vi "ProjetoTASCA.vi"(11 "Measurement Time (s)":sgl=1.0) -> (1 "Coincidences":u32=9, 2 "Count 1":u32=42663, 3 "Count 0":u32=44178)   [LabVIEW 2013]
uses:
  <vilib>/eio/EIONode/EIONode.xnode
  <vilib>/rvi/eio/common/nirviEmuTemplateMethod_errors.vi
  <vilib>/Platform/TimedLoop/XDataNode/XDataNode.xnode
  <vilib>/Platform/TimedLoop/XDataNode/timing_clust.ctl
  <vilib>/Platform/TimedLoop/XDataNode/XDNodeRunTimeDep.lvlib
  <vilib>/Platform/TimedLoop/XDataNode/wakeup.ctl
  <vilib>/Platform/TimedLoop/XDataNode/nitl_modes.ctl
panel:
  out "execution rate out":u32
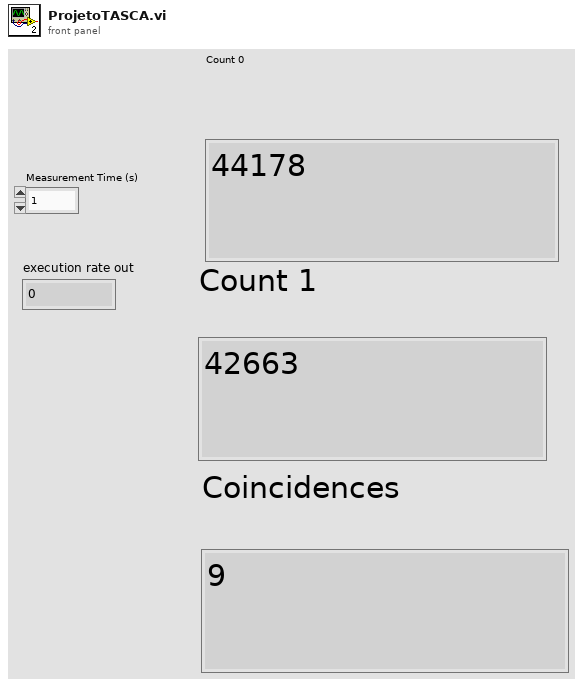
[diagram p1: front panel]
types:
  T1 = typedef "XDNodeRunTimeDep.lvlib/timing_clust.ctl" = cluster{"Expected End [f-1]":u64, "Actual End [f-1]":u64, "Finished Late? [f-1]":bool, "Expected End [i-1]":u64, "Actual End [i-1]":u64, "Finished Late? [i-1]":bool, "Expected Start [i]":u64, "Actual Start [i]":u64, "Expected Start [f]":u64, "Actual Start [f]":u64, "Source Name":string, "Structure Name":string, "Period":i64, "Deadline":i64, "Offset":i64, "Start":i64, "Priority":i32, "Timeout":i32, "Mode":T2, "Wakeup Reason":T3, "Error":errorcluster, "Source Type":string, "Secondary Source Type":string, "Global End Time":u64, "Global Start Time":u64, "Frame Duration":u64, "Iteration Duration":u64, "Assigned CPU":i32, "I/O Scan Engine Mode":u32}
  T2 = typedef "XDNodeRunTimeDep.lvlib/nitl_modes.ctl" = enum32{"No Change", "Process missed periods, maintain original phase", "Discard missed periods, maintain original phase", "Process missed periods, ignore original phase", "Discard missed periods, ignore original phase"}
  T3 = typedef "XDNodeRunTimeDep.lvlib/wakeup.ctl" = enum32{"Normal", "Aborted", "Asynchronous wakeup", "Timing source error", "Timed loop error", "Timeout"}
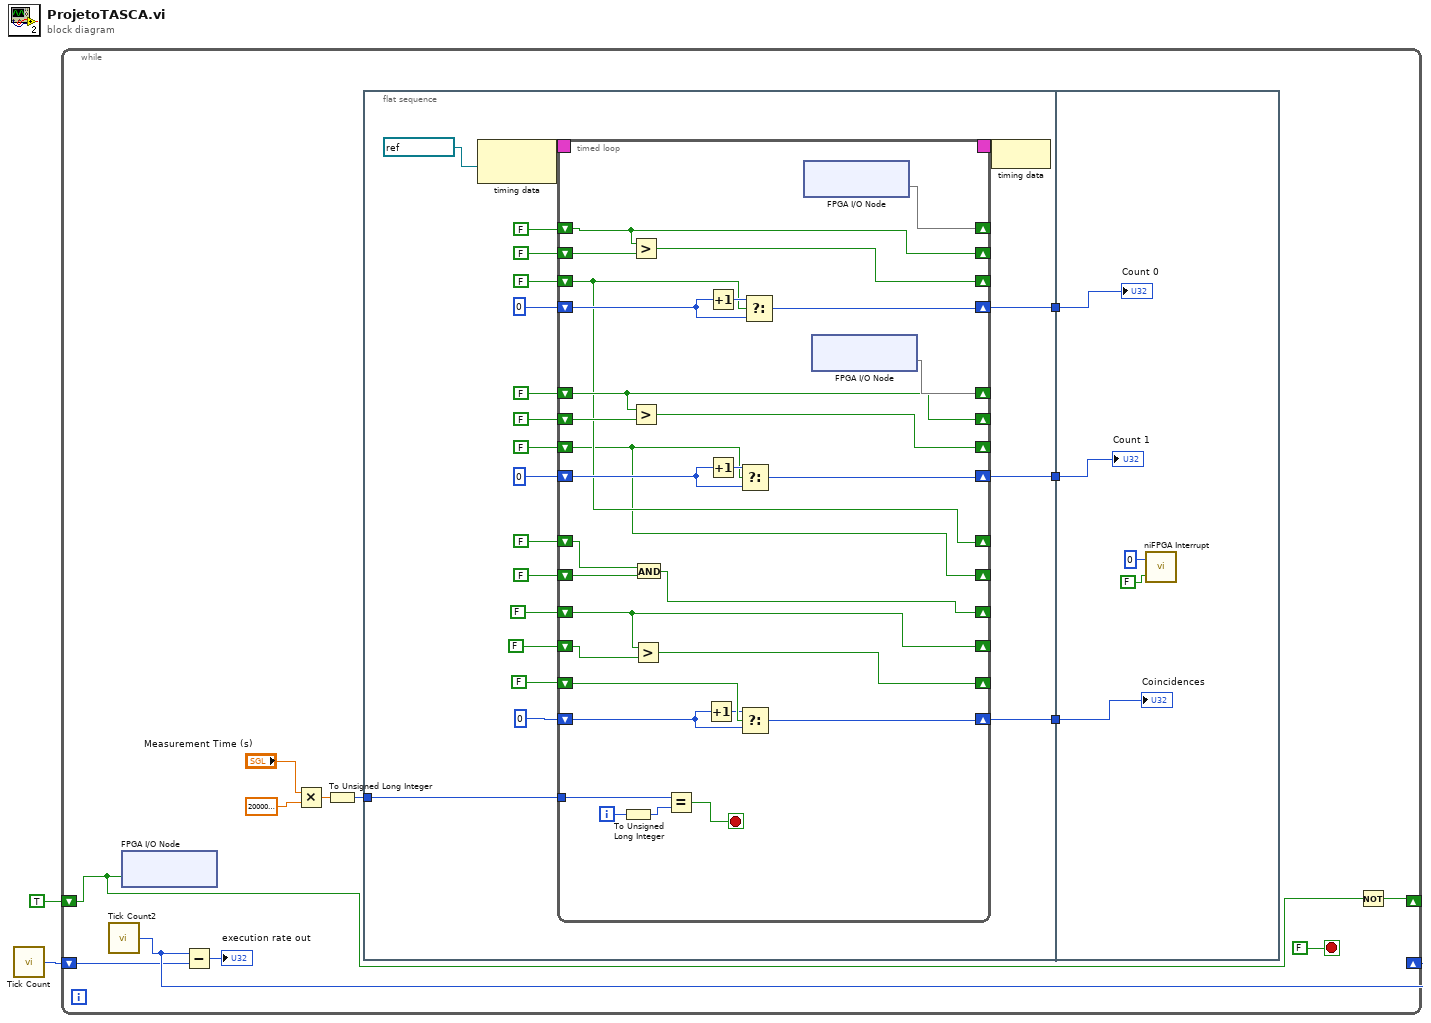
[diagram p0: block diagram]
diagram:
  n1 = call "Tick Count"() -> ("Tick Count(Ticks)"=w2:u32)
  n2 = while {
    shift-right: [w8] -> _
    shift-left: w2 -> [w7]
    shift-right: [w4] -> _
    shift-left: TRUE -> [w3]
    stop <- FALSE stop-if-true
    n3 = call "Tick Count2"() -> ("Tick Count(Ticks)"=w8:u32)
    n4 = xnode "FPGA I/O Node"("FPGA LED"=w3) -> ()  [unwired: 1 in, 1 out]
    n5 = Subtract(x=w8, y=w7) -> (x-y=→"execution rate out":u32)
    n6 = Multiply(x="Measurement Time (s)", y=sgl 200000000.0) -> (x*y=w11:sgl)
    n7 = To Unsigned Long Integer(number=w11) -> (unsigned 32bit integer=w5:u32)
    n8 = flat-sequence {
      tunnel: [w19] -> w15
      tunnel: [w18] -> w14
      tunnel: [w17] -> w13
      tunnel: w5 -> [w16]
      tunnel: w15 -> [w75]
      tunnel: w14 -> [w77]
      tunnel: w13 -> [w76]
      frame #0 {
        n9 = node-c288(refnum<k21> "200MHz" ("Source Name")) -> (w36:T1)
        n10 = timed-loop {
          timing: w36 -> [_]
          timing-out: [_] -> w35
          shift-right: [w66] -> _
          shift-left: FALSE ("Mod1/DIO0") -> [w65]
          shift-right: [w65] -> _
          shift-left: FALSE ("Mod1/DIO0") -> [w64]
          shift-right: [w63] -> _
          shift-left: FALSE ("Mod1/DIO0") -> [w40]
          shift-right: [w60] -> w19
          shift-left: u32 0 -> [w61]
          shift-right: [w59] -> _
          shift-left: FALSE ("Mod1/DIO1") -> [w58]
          shift-right: [w58] -> _
          shift-left: FALSE ("Mod1/DIO1") -> [w57]
          shift-right: [w41] -> _
          shift-left: FALSE -> [w39]
          shift-right: [w56] -> w17
          shift-left: u32 0 -> [w54]
          shift-right: [w40] -> _
          shift-left: FALSE ("Mod1/DIO0") -> [w53]
          shift-right: [w39] -> _
          shift-left: FALSE -> [w52]
          shift-right: [w51] -> _
          shift-left: FALSE -> [w48]
          shift-right: [w48] -> _
          shift-left: FALSE -> [w50]
          shift-right: [w49] -> _
          shift-left: FALSE -> [w47]
          shift-right: [w46] -> w18
          shift-left: u32 0 -> [w45]
          tunnel: w16 -> [w37]
          i -> [w43]
          stop <- w38 stop-if-true
          n11 = To Unsigned Long Integer(number=w43) -> (unsigned 32bit integer=w42:u32)
          n12 = Greater?(x=w65, y=w64) -> (0:w63:bool)
          n13 = Greater?(x=w58, y=w57) -> (0:w41:bool)
          n14 = Greater?(x=w48, y=w50) -> (0:w49:bool)
          n15 = And(x=w53, y=w52) -> (x .and. y?=w51:bool)
          n16 = Equal?(x=w37, y=w42) -> (x = y?=w38:bool)
          n17 = Increment(x=w45) -> (x+1=w44:u32)
          n18 = Increment(x=w61) -> (x+1=w62:u32)
          n19 = Increment(x=w54) -> (x+1=w55:u32)
          n20 = Select(t=w55, s=w39, f=w54) -> (s? t:f=w56:u32)
          n21 = Select(t=w44, s=w47, f=w45) -> (s? t:f=w46:u32)
          n22 = Select(t=w62, s=w40, f=w61) -> (s? t:f=w60:u32)
          n23 = xnode "FPGA I/O Node"() -> ("Mod1/DIO0"=w66)  [unwired: 1 in, 1 out]
          n24 = xnode "FPGA I/O Node"() -> ("Mod1/DIO1"=w59)  [unwired: 1 in, 1 out]
        }
        n25 = node-c288(w35) -> ()
      }
      frame #1 {
        n26 = call <vilib>:"niFPGA Interrupt.vi"("Wait Until Cleared (F)"=FALSE, "IRQ Number (0)"=u8 0) -> ()  [unwired: 1 in]
        "Coincidences" <- w77
        "Count 1" <- w76
        "Count 0" <- w75
      }
    }
    n27 = Not(x=w3) -> (.not. x?=w4:bool)
  }
